vi "SubStabilize.vi"(8 "error in (no error)":errorcluster, 10 "Rectangle":T1 {"Rotation" min=-90.0 max=90.0 step=1.0 format="%.2f"; "Left" scale=0.0..1024.0; "Right" scale=0.0..1024.0}, 11 "path":path) -> (0 "error out":errorcluster)   [LabVIEW 2017]
uses:
  <vilib>/vision/NI_Vision_Development_Module.lvlib
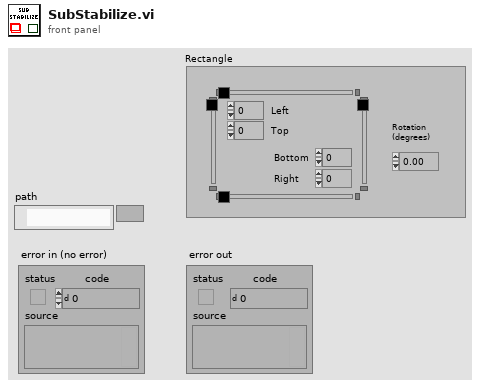
[diagram p1: front panel]
types:
  T1 = typedef "IMAQ Rectangle" = cluster{"Left":i32, "Top":i32, "Right":i32, "Bottom":i32, "Rotation":dbl}
  T2 = typedef "IMAQ AVI2 Refnum.ctl" = refnum<k20>
  T3 = typedef "IMAQ Image.ctl" = refnum<image>
  T4 = cluster{"Width":u32, "Height":u32, "Frames Per Second":u32, "Codec":string, "Has Data":bool}
  T5 = typedef "ROI Descriptor" = cluster{"Global Rectangle":i32[], "Contours":cluster{"ID":enum32{"External", "Internal"}, "Type":u32, "Coordinates":i32[]}[]}
  T6 = cluster{"Position":cluster{"x":sgl, "y":sgl}, "Angle":sgl, "Scale":sgl, "Score":sgl, "Bounding Box":cluster{"x":sgl, "y":sgl}[]}[]
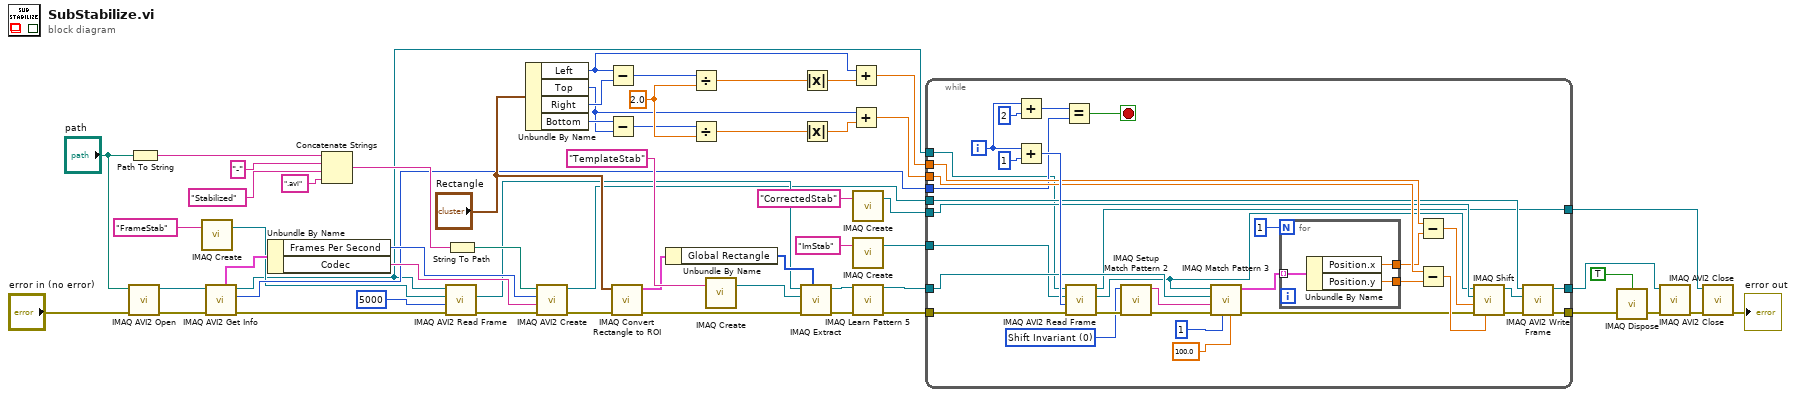
[diagram p0: block diagram]
diagram:
  w50 = 2.0 ("y")
  n1 = call "IMAQ AVI2 Open"("error in (no error)"="error in (no error)", "AVI File Path"="path") -> ("error out"=w17:errorcluster, "AVI Refnum"=w18:T2)  [unwired: 8 in]
  n2 = Path To String(path="path") -> (string=w27:string)
  n3 = call "IMAQ Create"("Image Name"="FrameStab") -> ("New Image"=w11:T3)  [unwired: 4 in, 1 out]
  n4 = call "IMAQ AVI2 Get Info"("error in (no error)"=w17, "AVI Refnum"=w18) -> ("error out"=w4:errorcluster, "Number of Frames"=w13:u32, "AVI Refnum (duplicate)"=w7:T2, "Frame Data"=w15:T4)  [unwired: 5 in, 1 out]
  n5 = Unbundle By Name(w15) -> ("Frames Per Second"=w21:u32, "Codec"=w20:string)
  n6 = Concatenate Strings(w27, "-" ("string"), "Stabilized" ("string"), ".avi" ("string")) -> (w24:string)
  n7 = call "IMAQ AVI2 Read Frame"("error in (no error)"=w4, "Frame Number"=u32 5000, "Image"=w11, "AVI Refnum"=w7) -> ("error out"=w5:errorcluster, "Image Out"=w10:T3)  [unwired: 5 in, 1 out]
  n8 = String To Path(string=w24) -> (path=w22:path)
  n9 = Unbundle By Name("Rectangle") -> ("Left"=w45:i32, "Top"=w44:i32, "Right"=w47:i32, "Bottom"=w46:i32)
  n10 = call "IMAQ AVI2 Create"("error in (no error)"=w5, "Codec"=w20, "Frames Per Second"=w21, "AVI Path"=w22) -> ("error out"=w6:errorcluster, "AVI Refnum"=w8:T2)  [unwired: 6 in]
  n11 = Subtract(x=w45, y=w47) -> (x-y=w49:i32)
  n12 = Subtract(x=w46, y=w44) -> (x-y=w48:i32)
  n13 = call "IMAQ Convert Rectangle to ROI"("error in (no error)"=w6, "Rectangle"="Rectangle") -> ("error out"=w55:errorcluster, "ROI Descriptor"=w54:T5)  [unwired: 7 in]
  n14 = Unbundle By Name(w54) -> ("Global Rectangle"=w53:i32[])
  n15 = Divide(x=w49, y=w50) -> (x/y=w41:dbl)
  n16 = Divide(x=w48, y=w50) -> (x/y=w39:dbl)
  n17 = call "IMAQ Create"("Image Name"="TemplateStab") -> ("New Image"=w56:T3)  [unwired: 4 in, 1 out]
  n18 = call "IMAQ Extract"("Optional Rectangle"=w53, "error in (no error)"=w55, "Image Dst"=w56, "Image Src"=w10) -> ("error out"=w51:errorcluster, "Image Dst Out"=w52:T3)  [unwired: 6 in]
  n19 = Absolute Value(x=w41) -> (abs(x)=w40:dbl)
  n20 = Absolute Value(x=w39) -> (abs(x)=w38:dbl)
  n21 = Add(x=w45, y=w40) -> (x+y=w43:dbl)
  n22 = Add(x=w44, y=w38) -> (x+y=w42:dbl)
  n23 = call "IMAQ Create"("Image Name"="CorrectedStab") -> ("New Image"=w31:T3)  [unwired: 4 in, 1 out]
  n24 = call "IMAQ Create"("Image Name"="ImStab") -> ("New Image"=w33:T3)  [unwired: 4 in, 1 out]
  n25 = call "IMAQ Learn Pattern 5"("Image"=w52, "error in (no error)"=w51) -> ("Template Image Out"=w37:T3, "error out"=w36:errorcluster)  [unwired: 11 in, 1 out]
  n26 = while {
    tunnel: w37 -> [w75]
    tunnel: w43 -> [w83]
    tunnel: w42 -> [w81]
    tunnel: w8 -> [w79]
    tunnel: w36 -> [w71]
    tunnel: [w73] -> w35
    tunnel: w33 -> [w72]
    tunnel: w31 -> [w70]
    tunnel: [w69] -> w29
    tunnel: w13 -> [w62]
    tunnel: w7 -> [w61]
    tunnel: [w58] -> w1
    i -> [w89]
    stop <- w86 stop-if-true
    w66 = u16 0 items=["Shift Invariant", "Rotation Invariant"] ("Match Mode")
    n27 = Add(x=w89, y=2) -> (x+y=w87:i32)
    n28 = Add(x=w89, y=1) -> (x+y=w90:i32)
    n29 = Equal?(x=w87, y=w62) -> (x = y?=w86:bool)
    n30 = call "IMAQ AVI2 Read Frame"("error in (no error)"=w71, "Frame Number"=w90, "Image"=w72, "AVI Refnum"=w61) -> ("error out"=w78:errorcluster, "Image Out"=w64:T3, "AVI Refnum (duplicate)"=w58:T2)  [unwired: 5 in]
    n31 = call "IMAQ Setup Match Pattern 2"("error in (no error)"=w78, "Match Mode"=w66) -> ("error out"=w77:errorcluster, "Match Pattern Setup Data"=w76:string)  [unwired: 8 in]
    n32 = call "IMAQ Match Pattern 3"("Minimum Match Score"=sgl 100.0, "Number of Matches Requested"=1, "error in (no error)"=w77, "Match Pattern Setup Data"=w76, "Template Image"=w75, "Image"=w64) -> ("error out"=w63:errorcluster, "Matches"=w85:T6)  [unwired: 3 in, 1 out]
    n33 = for {
      N: 1 -> [_]
      tunnel: w85 -> [w94] mode=indexing
      tunnel: [w93] -> w68
      tunnel: [w92] -> w67
      n34 = Unbundle By Name(w94) -> ("Position.x"=w93:sgl, "Position.y"=w92:sgl)
    }
    n35 = Subtract(x=w83, y=w68) -> (x-y=w82:dbl)
    n36 = Subtract(x=w81, y=w67) -> (x-y=w80:dbl)
    n37 = call "IMAQ Shift"("YOffset"=w80, "error in (no error)"=w63, "XOffset"=w82, "Image Dst"=w70, "Image Src"=w64) -> ("error out"=w60:errorcluster, "Image Dst Out"=w59:T3)  [unwired: 5 in]
    n38 = call "IMAQ AVI2 Write Frame"("error in (no error)"=w60, "Image"=w59, "AVI Refnum"=w79) -> ("error out"=w69:errorcluster, "AVI Refnum (duplicate)"=w73:T2)  [unwired: 6 in, 1 out]
  }
  n39 = call "IMAQ Dispose"("All Images? (No)"=TRUE, "error in (no error)"=w29) -> ("error out"=w28:errorcluster)  [unwired: 4 in]
  n40 = call "IMAQ AVI2 Close"("error in (no error)"=w28, "AVI Refnum"=w35) -> ("error out"=w3:errorcluster)  [unwired: 9 in]
  n41 = call "IMAQ AVI2 Close"("error in (no error)"=w3, "AVI Refnum"=w1) -> ("error out"=→"error out":errorcluster)  [unwired: 9 in]
